vi "CSP_estimateCovarianceMatrix.vi"(8 "error in (no error)":errorcluster, 10 "Processing file":refnum<vi>, 11 "FilePaths":path[](array[path])) -> (0 "error out":errorcluster, 2 "Mean Trial":dbl[][](array[numeric]), 3 "Covariance Matrix":T1)   [LabVIEW 2016, in "Spatial Pattern Filter.lvlib"]
uses:
  Spatial Pattern Filter.lvlib
  <vilib>/Analysis/Matrix/Datatypes/RealMatrix.ctl
  _XML_EEG_File_Parser/_vlib/XML_EEG_File.lvclass
  <vilib>/xml/Load XML File.vi
  <vilib>/addons/Time Series Analysis/Statistical Analysis.llb/TSA Covariance (Waveform).vi
  <vilib>/Analysis/Matrix/Numeric/Conversions/Array To Matrix - RA2.vi
  <vilib>/Analysis/Matrix/Numeric/Add/Add - RM,RM.vi
  <vilib>/xml/NI_XML.lvlib
  <vilib>/Analysis/Matrix/NI_Matrix.lvlib
  <vilib>/addons/_Advanced Signal Processing/NI_AdvSigProcTSA.lvlib
panel:
  # "This VI is a part of BCI Design library, http://www.ru-bci.org \nCopyright © 2020, Sotnikov Peter, All rights reserved. License: CC BY-NC 4.0"
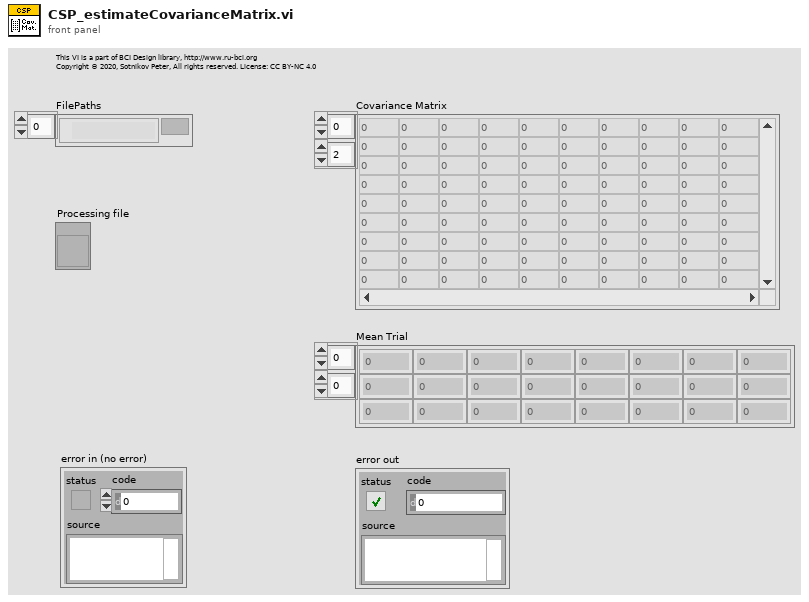
[diagram p1: front panel]
types:
  T1 = typedef "NI_Matrix.lvlib/RealMatrix.ctl" = dbl[][]
  T2 = typedef "XML_EEG_File_Parser.lvlib/XML_EEG_Header.ctl" = cluster{"Attributes":cluster{"ChannelDataType":string, "NumberOfChannels":i32, "SampleRateHz":dbl, "MarkerChannel":i32}, "Body":cluster{"PatientSpecificData":string, "NumberOfDatasets":i32, "Channels":string[]}}
  T3 = typedef "XML_EEG_File_Parser.lvlib/XML_EEG_Dataset.ctl" = cluster{"Attributes":cluster{"NumberOfSamples":i32, "StartDateTime":timestamp}, "Body":cluster{"MarkerValue":string, "Channels":waveform(dbl)[]}}
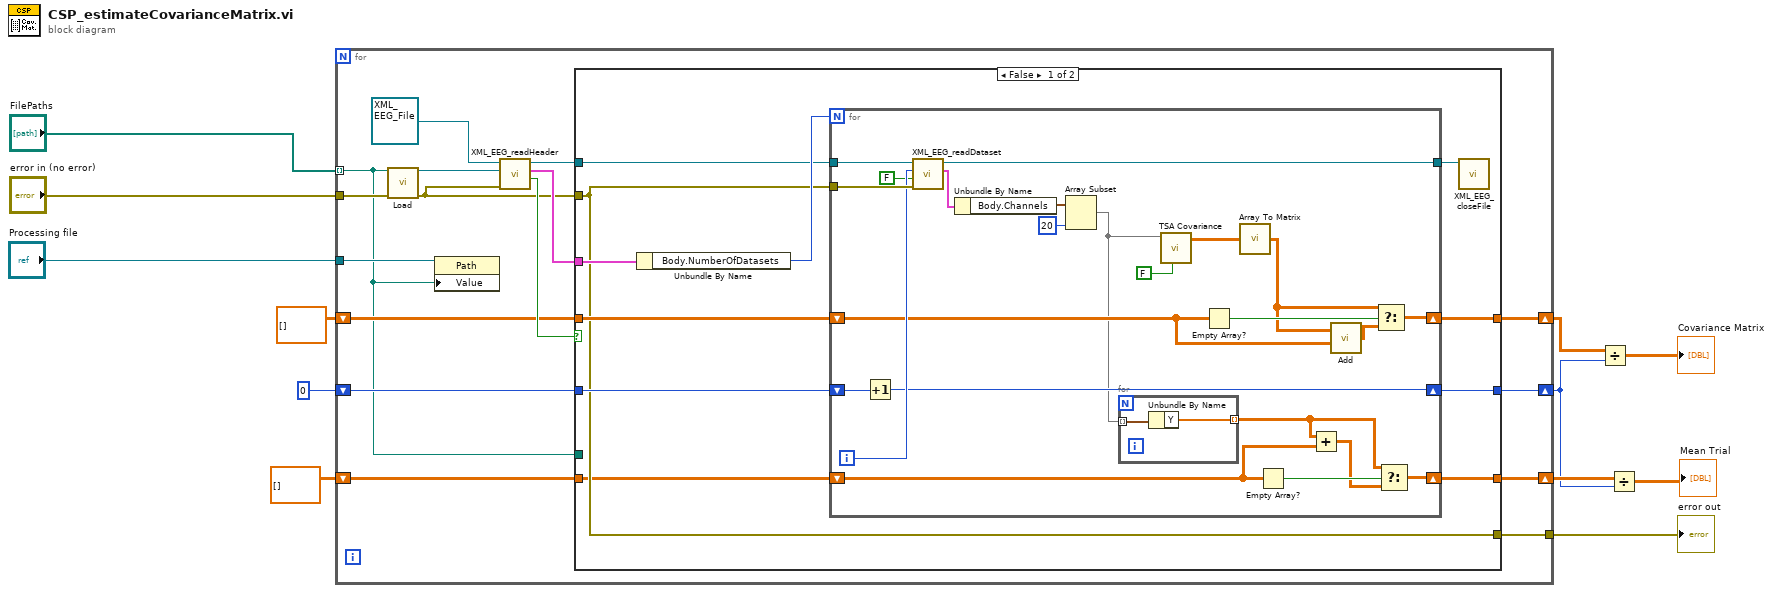
[diagram p0: block diagram]
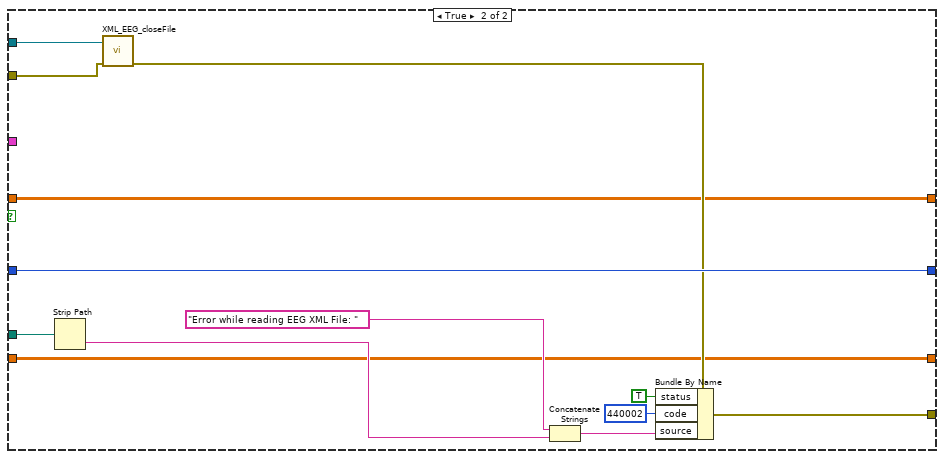
[diagram p2: hidden frame]
diagram:
  n1 = for {
    tunnel: "error in (no error)" -> [w28]
    shift-right: [w20] -> w2
    shift-left: 0 -> [w21]
    tunnel: "FilePaths" -> [w15] mode=indexing
    shift-right: [w18] -> w9
    shift-left: T1 [] ("A + B") -> [w19]
    tunnel: [w17] -> w7
    tunnel: "Processing file" -> [w16]
    shift-right: [w13] -> w3
    shift-left: dbl[][] [] -> [w14]
    n2 = call-poly <vilib>:"Load.vi"("path to XML document"=w15, "error in (no error)"=w28) -> ("DOM document out"=w27:refnum<k20>, "error out"=w22:errorcluster)  [unwired: 11 in, 1 out]
    n3 = property class="Path"(reference=w16, "Value"=w15) -> ()  [unwired: 1 in, 2 out]
    n4 = call "XML_EEG_readHeader.vi"("error in (no error)"=w22, "DOM document in"=w27, "XML_EEG_Class in"=refnum<class "XML_EEG_File.lvclass"> refnum ("XML_EEG_File_Parser.lvlib:XML_EEG_File.lvclass")) -> ("Errors?"=w25:bool, "XML Header out"=w24:T2, "XML_EEG_Class out"=w23:refnum<class "XML_EEG_File.lvclass">)  [unwired: 6 in]
    n5 = case shown="False" w25 {
      tunnel: w24 -> [w39 _]
      tunnel: w23 -> [w37 w77]
      tunnel: w22 -> [w31 w76]
      tunnel: w21 -> [w35 w75]
      tunnel: [w34 w75] -> w20
      tunnel: w19 -> [w33 w70]
      tunnel: [w32 w70] -> w18
      tunnel: [w31 w71] -> w17
      tunnel: w15 -> [_ w69]
      tunnel: w14 -> [w30 w65]
      tunnel: [w29 w65] -> w13
      frame False {
        n6 = Unbundle By Name(w39) -> ("Body.NumberOfDatasets"=w38:i32)
        n7 = for {
          N: w38 -> [_]
          tunnel: w37 -> [w62]
          tunnel: w31 -> [w61]
          tunnel: [w43] -> w36
          shift-right: [w56] -> w34
          shift-left: w35 -> [w57]
          shift-right: [w55] -> w32
          shift-left: w33 -> [w53]
          shift-right: [w48] -> w29
          shift-left: w30 -> [w46]
          i -> [w60]
          n8 = Increment(x=w57) -> (x+1=w56:i32)
          n9 = call "XML_EEG_readDataset.vi"("error in (no error)"=w61, "Add offset?"=FALSE, "DatasetNumber"=w60, "XML_EEG_File in"=w62) -> ("XML Dataset out"=w58:T3, "XML_EEG_File out"=w43:refnum<class "XML_EEG_File.lvclass">)  [unwired: 5 in, 1 out]
          n10 = Unbundle By Name(w58) -> ("Body.Channels"=w42:waveform(dbl)[])
          n11 = Array Subset(array=w42, length=20) -> (w41:waveform(dbl)[])  [unwired: 1 in]
          n12 = for {
            tunnel: w41 -> [w64] mode=indexing
            tunnel: [w63] -> w44 mode=indexing
            n13 = Unbundle By Name(w64) -> ("Y"=w63:dbl[])
          }
          n14 = call-poly <vilib>:"TSA Covariance.vi"("normalized? (F)"=FALSE, "Xt"=w41) -> ("covariance"=w50:dbl[][])  [unwired: 8 in, 1 out]
          n15 = Empty Array?(array=w53) -> (empty?=w54:bool)
          n16 = call-poly <vilib>:"Array To Matrix.vi"("Real 2D Array"=w50) -> ("Real Matrix"=w49:T1)
          n17 = Empty Array?(array=w46) -> (empty?=w47:bool)
          n18 = Add(x=w44, y=w46) -> (x+y=w45:dbl[][])
          n19 = call-poly <vilib>:"Add.vi"("Real Matrix B"=w53, "Real Matrix A"=w49) -> ("A + B"=w52:T1)
          n20 = Select(t=w49, s=w54, f=w52) -> (s? t:f=w55:T1)
          n21 = Select(t=w44, s=w47, f=w45) -> (s? t:f=w48:dbl[][])
        }
        n22 = call "XML_EEG_closeFile.vi"("XML_EEG_File.lvclass"=w36) -> ()  [unwired: 10 in, 1 out]
      }
      frame True {
        n23 = Strip Path(path=w69) -> (name=w66:string)  [unwired: 1 out]
        n24 = call "XML_EEG_closeFile.vi"("error in (no error)"=w76, "XML_EEG_File.lvclass"=w77) -> ("error out"=w74:errorcluster)  [unwired: 9 in]
        n25 = Concatenate Strings("Error while reading EEG XML File: " ("source"), w66) -> (w68:string)
        n26 = Bundle By Name(cluster=w74, "status"=TRUE, "code"=440002, "source"=w68) -> (w71:errorcluster)
      }
    }
  }
  "error out" <- w7
  n27 = Divide(x=w9, y=w2) -> (x/y=→"Covariance Matrix":T1)
  n28 = Divide(x=w3, y=w2) -> (x/y=→"Mean Trial":dbl[][])
